vi "Fit.vi"(8 "error in (no error)":errorcluster caption="entrée d'erreur (pas d'erreur)", 9 "y":string[][](array[string]), 10 "X":string[][](array[string]), 11 "PowerTransformer.lvclass":refnum<class "PowerTransformer.lvclass">) -> (0 "error out":errorcluster caption="sortie d'erreur", 2 "String Data":string, 3 "PowerTransformer.lvclass":refnum<class "PowerTransformer.lvclass">)   [LabVIEW 2020, in "PowerTransformer.lvclass"]
doc: "Estimate the optimal parameter lambda for each feature.\n\nThe optimal lambda parameter for minimizing skewness is estimated on each feature independently using maximum likelihood.\n\nReturns : \n\n- String : OK"
uses:
  PowerTransformer.lvclass
  PowerTransformer.lvclass/PowerTransformer.ctl
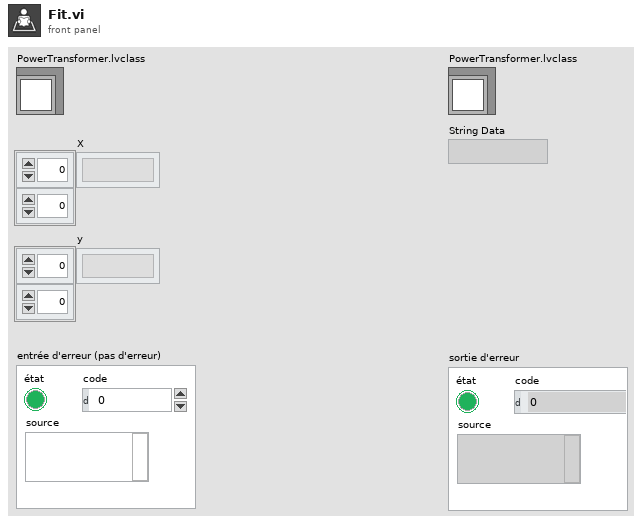
[diagram p1: front panel]
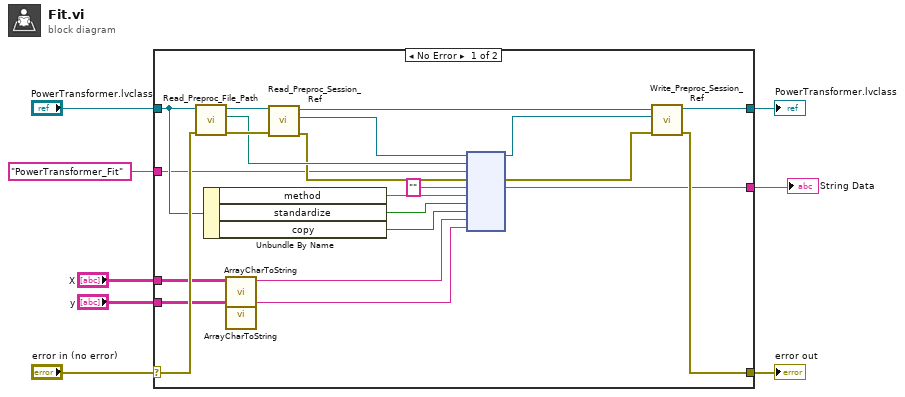
[diagram p0: block diagram]
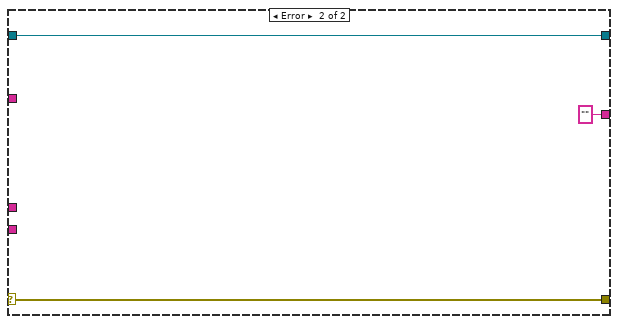
[diagram p2: hidden frame]
diagram:
  n1 = case shown="No Error" "error in (no error)" {
    selector: "error in (no error)" -> [w18 w33]
    tunnel: [w16 w33] -> w7
    tunnel: [w17 w32] -> w5
    tunnel: "PowerTransformer.lvclass" -> [w15 w32]
    tunnel: "PowerTransformer_Fit" ("Fonction") -> [w14 _]
    tunnel: [w13 ""] -> w3
    tunnel: "X" -> [w12 _]
    tunnel: "y" -> [w11 _]
    frame No Error {
      n2 = call-dynamic "Read_Preproc_File_Path.vi"("error in (no error)"=w18, "Python in"=w15) -> ("error out"=w29:errorcluster, "File_Path"=w26:path, "Python out"=w30:refnum<class "PowerTransformer.lvclass">)  [unwired: 7 in]
      n3 = Unbundle By Name(w15) -> ("method"=w21:string, "standardize"=w20:bool, "copy"=w19:bool)
      n4 = call "ArrayCharToString.vi"("TAB"=w12) -> ("Instruction"=w10:string)  [unwired: 10 in]
      n5 = call "ArrayCharToString.vi"("TAB"=w11) -> ("Instruction"=w9:string)  [unwired: 10 in]
      n6 = call-dynamic "Read_Preproc_Session_Ref.vi"("error in (no error)"=w29, "Python in"=w30) -> ("error out"=w25:errorcluster, "Session_ref"=w27:refnum<k35>, "Python out"=w28:refnum<class "PowerTransformer.lvclass">)  [unwired: 7 in]
      n7 = node(w27, w26, w14, w25, "", w21, w20, w19, w10, w9) -> (w23:refnum<k35>, w24:errorcluster, w13:string)  [unwired: 5 in, 2 out]
      n8 = call-dynamic "Write_Preproc_Session_Ref.vi"("error in (no error)"=w24, "Session_ref"=w23, "Python in"=w28) -> ("error out"=w16:errorcluster, "Python out"=w17:refnum<class "PowerTransformer.lvclass">)  [unwired: 7 in]
    }
    frame Error {
    }
  }
  "error out" <- w7
  "PowerTransformer.lvclass" <- w5
  "String Data" <- w3
